vi "Actor Core.vi"(8 "error in":errorcluster, 11 "Pane Relief Main UI in":refnum<class "Pane Relief Main UI.lvclass">) -> (0 "error out":errorcluster, 3 "Actor out":refnum<class "Actor.lvclass">)   [LabVIEW 2018, in "Pane Relief Main UI.lvlib" / "Pane Relief Main UI.lvclass"]
uses:
  <resource>/dialog/QuickDrop/plugins/PaneRelief/Classes/Pane Relief Main UI/Pane Relief Main UI/Pane Relief Main UI.lvclass
  C:/Program Files (x86)/National Instruments/LabVIEW 2018/vi.lib/MGI/Panel Manager/Panel Actor/Panel Actor/Panel Actor.lvclass
  <vilib>/ActorFramework/Actor/Actor.lvclass
  <resource>/dialog/QuickDrop/plugins/PaneRelief/Classes/Splitter Settings UI/Splitter Settings UI/Splitter Settings UI.lvclass
  <resource>/dialog/QuickDrop/plugins/PaneRelief/Classes/Pane Settings UI/Pane Settings UI/Pane Settings UI.lvclass
  <resource>/dialog/QuickDrop/plugins/PaneRelief/Classes/Pane Relief Main UI/Pane Relief Main UI/Pane Relief Main UI.lvclass/Pane Relief Main UI.ctl
  <vilib>/ActorFramework/Message Enqueuer/Message Enqueuer.lvclass/Message Enqueuer.ctl
  <resource>/dialog/QuickDrop/plugins/PaneRelief/Typedefs/UI Selections--Cluster.ctl
  <resource>/dialog/QuickDrop/plugins/PaneRelief/Typedefs/Point--Cluster.ctl
  <vilib>/Utility/sysdir.llb/System Directory Type.ctl
  <resource>/dialog/QuickDrop/plugins/PaneRelief/Classes/Panel Object/Panel Object.lvclass
  <resource>/dialog/QuickDrop/plugins/PaneRelief/Typedefs/Selection Colors--Cluster.ctl
  <vilib>/ActorFramework/Message Enqueuer/Enqueue.vi
  <vilib>/MGI/Panel Manager/Panel/Panel/Subpanel/Subpanel.lvclass
  C:/Program Files (x86)/National Instruments/LabVIEW 2018/vi.lib/MGI/Panel Manager/Panel/Panel/Panel.lvclass
  <vilib>/ActorFramework/Stop Msg/Stop Msg.lvclass
  C:/Program Files (x86)/National Instruments/LabVIEW 2018/vi.lib/ActorFramework/Message/Message.lvclass
  <resource>/dialog/QuickDrop/plugins/PaneRelief/Classes/Splitter/Splitter.lvclass
  C:/Program Files (x86)/National Instruments/LabVIEW 2018/resource/dialog/QuickDrop/plugins/PaneRelief/Classes/Panel Object/Panel Object.lvclass
  <resource>/dialog/QuickDrop/plugins/PaneRelief/Classes/Pane/Pane.lvclass
  <vilib>/MGI/Panel Manager/Panel/Panel/Subpanel/Subpanel.vi
  <vilib>/ActorFramework/Message Priority Queue/Priority Enqueue.vi
  <vilib>/MGI/Panel Manager/Panel Actor/Panel Actor/Panel Actor.lvclass
  <vilib>/MGI/Panel Manager/Panel/Panel.lvlib
panel:
  out "Nav Pic":picture
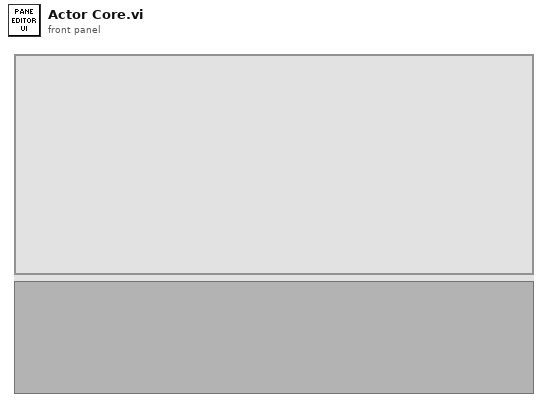
[diagram p1: front panel]
types:
  T1 = cluster{"Pnl Actor":refnum<event-registration>, "Event Registration Refnum":refnum<event-registration>}
  T2 = enum32{"Invalid", "Standard", "Closed", "Hidden", "Minimized", "Maximized"}
  T3 = enum32{"invalid app kind", "Development System", "Run Time System", "Student Edition", "Embedded LabVIEW", "Evaluation", "Custom"}
  T4 = typedef "LVPoint32TypeDef.ctl" = cluster{"Horizontal":i32, "Vertical":i32}
  T5 = typedef "Point--Cluster.ctl" = cluster{"Horizontal":i32, "Vertical":i32}
  T6 = typedef "UI Selections--Cluster.ctl" = cluster{"Mouse-over Idx":i32, "Selected Idx":i32}
  T7 = cluster{"Core":cluster{"Current VI Reference":refnum<vi>, "Close Panel on Exit?":bool}, "QD Launch VI Ref":refnum<vi>, "Panel Objects[]":refnum<class "Panel Object.lvclass">[], "UI Selections":T6, "Scale Factor":dbl, "Nav Pic Offset":T5, "Persistent Data Folder":path, "Persistent Data File":string}
  T8 = typedef "System Directory Type.ctl" = i32
  T9 = cluster{"Current VI Reference":refnum<vi>, "Close Panel on Exit?":bool}
  T10 = typedef "LVBoundsTypeDef.ctl" = cluster{"Width":u32, "Height":u32}
  T11 = typedef "LVPointTypeDef.ctl" = cluster{"Horizontal":i16, "Vertical":i16}
  T12 = typedef "Selection Colors--Cluster.ctl" = cluster{"Normal":u32, "Mouse-over":u32, "Selected":u32}
  T13 = typedef "imagedata.ctl" = cluster{"image type":i32, "image depth":i32, "image":u8[], "mask":u8[], "colors":u32[], "Rectangle":cluster{"left":i16, "top":i16, "right":i16, "bottom":i16}}
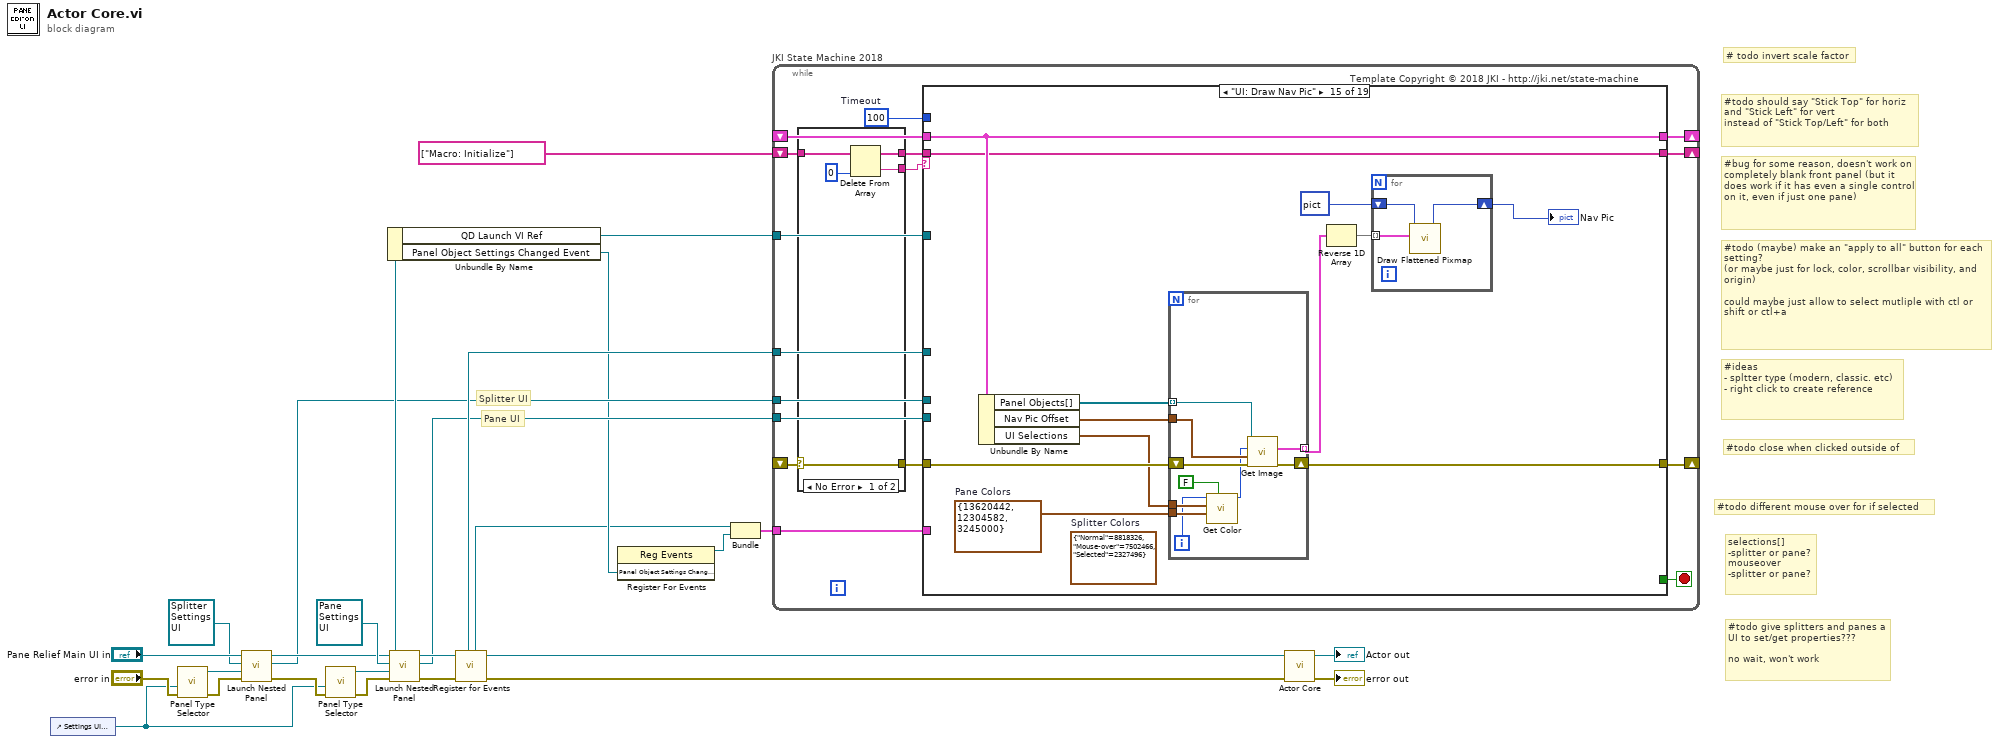
[diagram p0: block diagram]
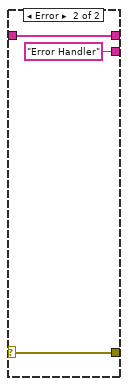
[diagram p2: hidden frame]
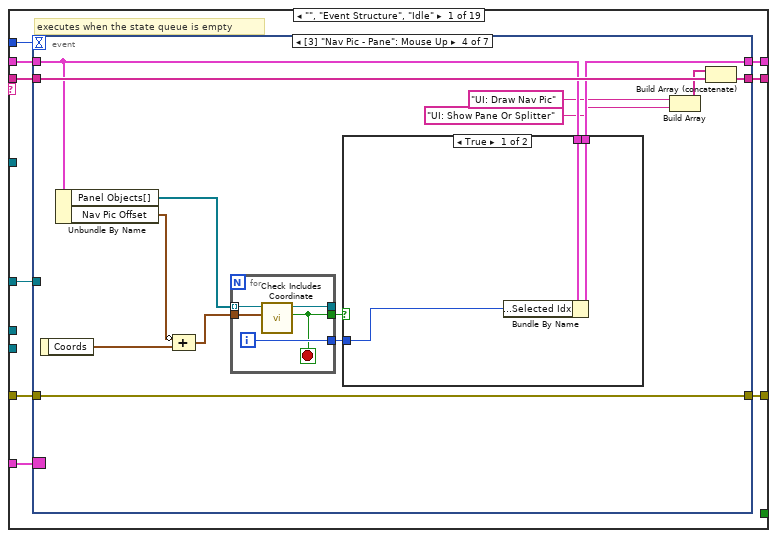
[diagram p3: hidden frame]
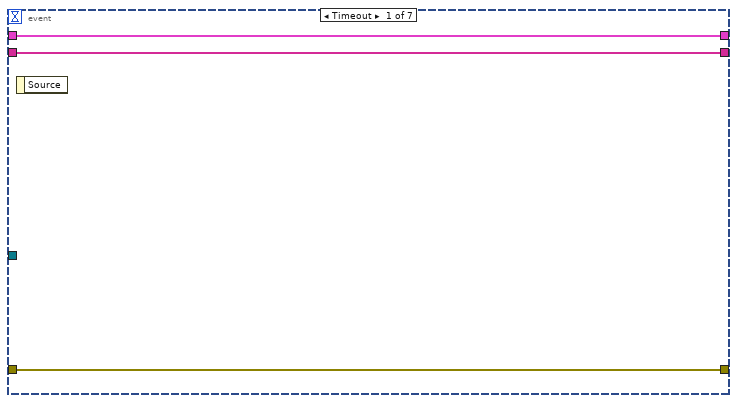
[diagram p4: hidden frame]
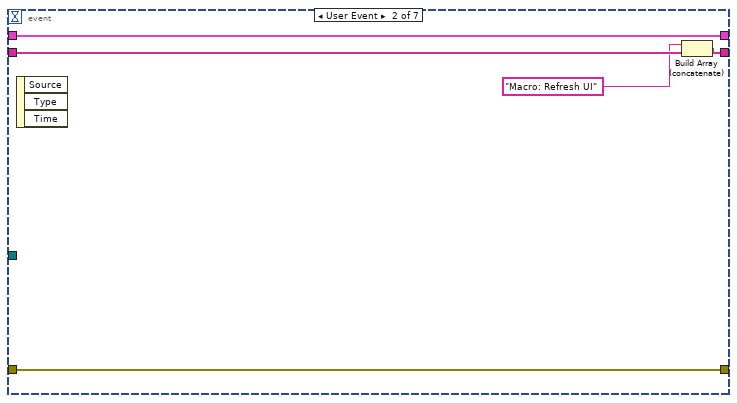
[diagram p5: hidden frame]
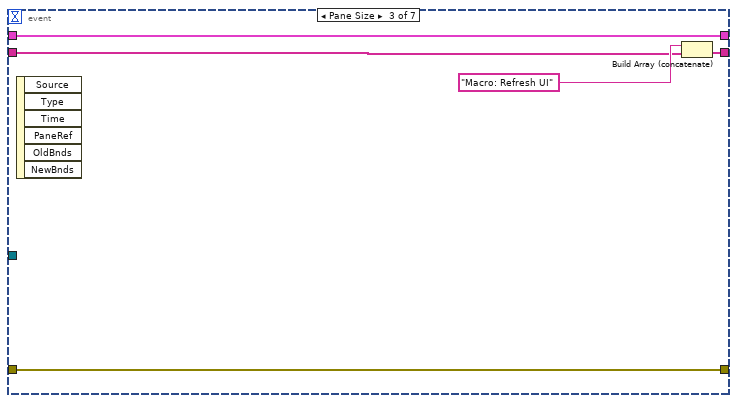
[diagram p6: hidden frame]
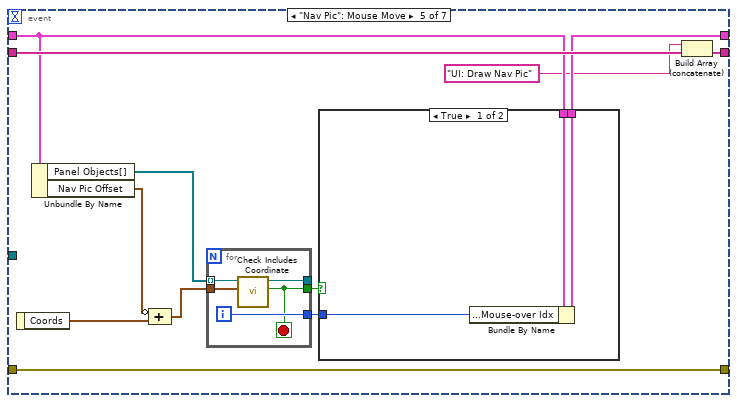
[diagram p8: hidden frame]
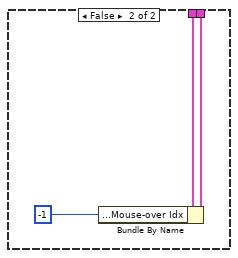
[diagram p9: hidden frame]
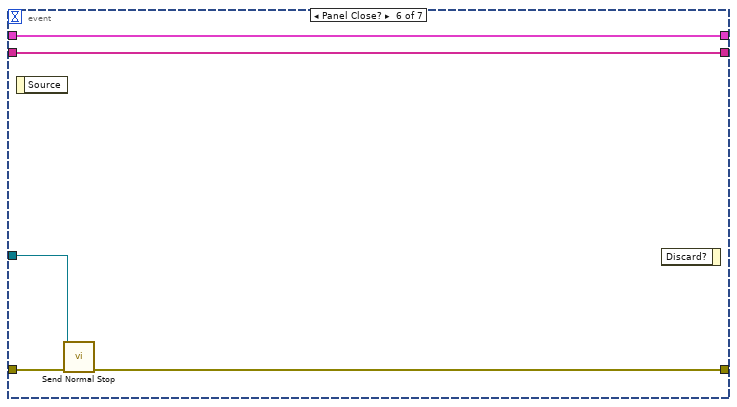
[diagram p10: hidden frame]
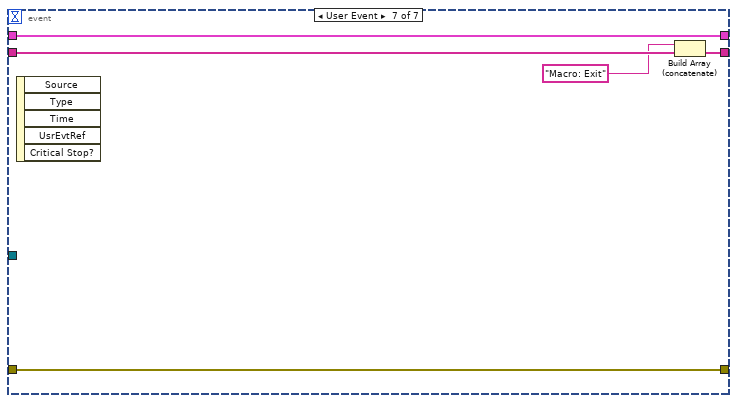
[diagram p11: hidden frame]
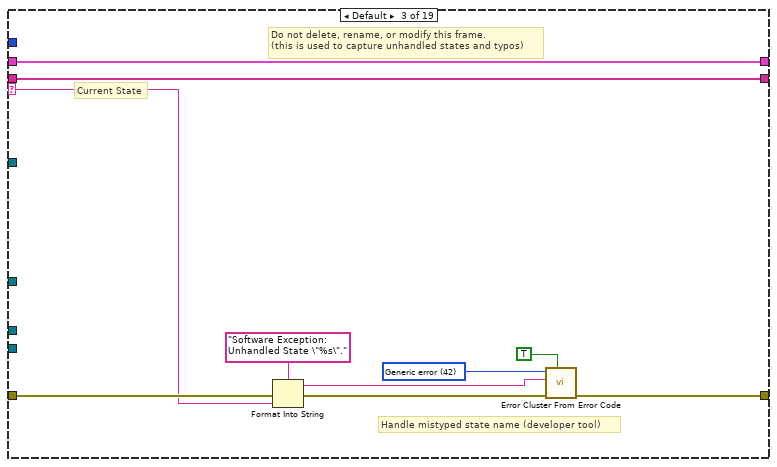
[diagram p13: hidden frame]
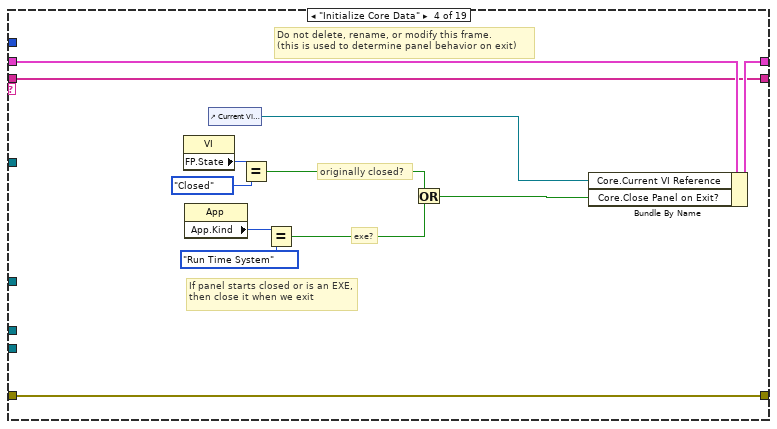
[diagram p14: hidden frame]
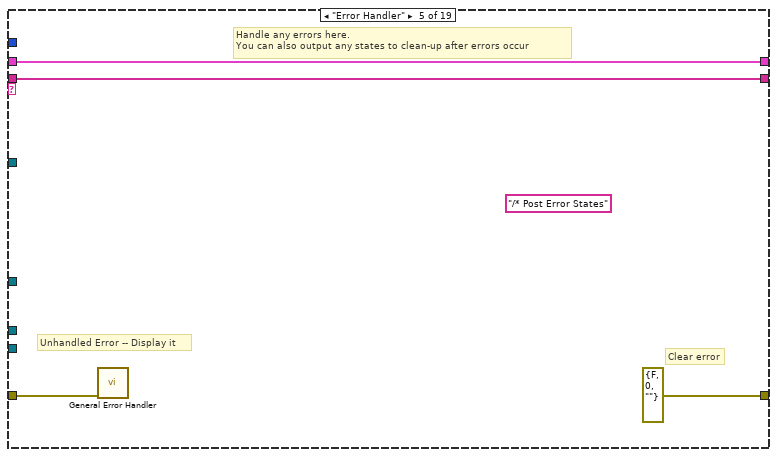
[diagram p15: hidden frame]
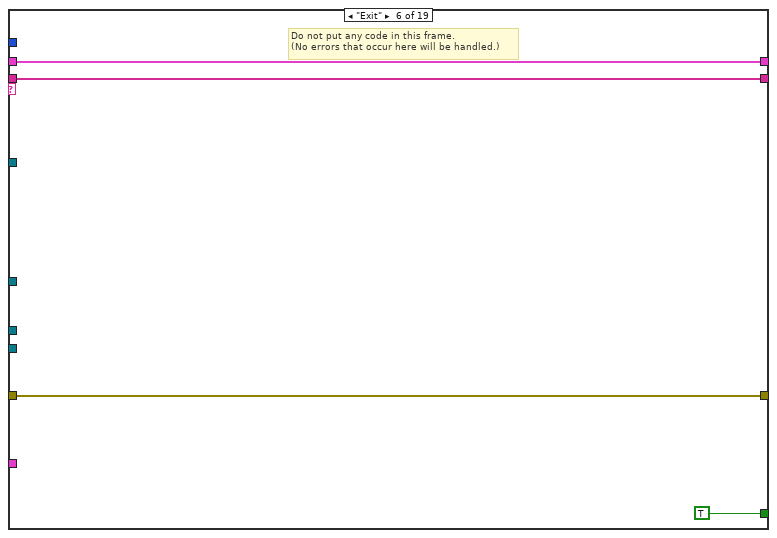
[diagram p16: hidden frame]
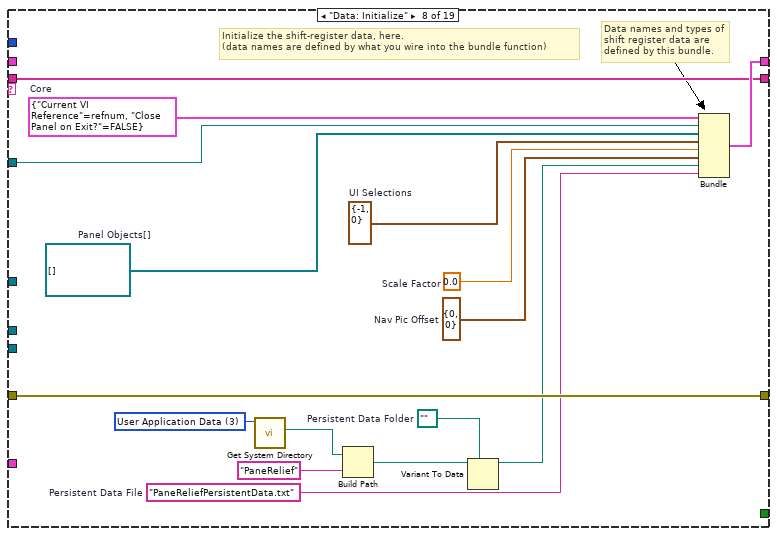
[diagram p18: hidden frame]
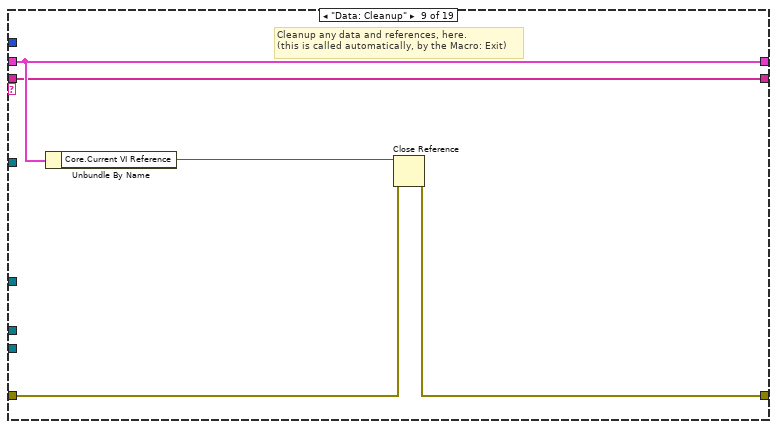
[diagram p19: hidden frame]
diagram:
  # "Pane UI"
  # "Splitter UI"
  # "#todo close when clicked outside of"
  # "#todo give splitters and panes a UI to set/get properties???\n\nno wait, won't work"
  # "# todo invert scale factor"
  # "selections[]\n-splitter or pane?\nmouseover\n-splitter or pane?"
  # "#todo different mouse over for if selected"
  # "#ideas\n- spltter type (modern, classic. etc)\n- right click to create reference"
  # "#todo (maybe) make an \"apply to all\" button for each setting?\n(or maybe just for lock, color, scrollbar visibility, and origin)\n\ncould maybe just allow to select mutliple with ctl or shift or ctl+a"
  # "#todo should say \"Stick Top\" for horiz and \"Stick Left\" for vert\ninstead of \"Stick Top/Left\" for both"
  # "#bug for some reason, doesn't work on completely blank front panel (but it does work if it has even a single control on it, even if just one pane)"
  n1 = control-ref of="Settings UI Subpanel"() -> (w12:refnum<vi>)
  n2 = call-poly <vilib>:"Panel Type Selector.vi"("Error In"="error in", "Sub Panel"=w12) -> ("Error Out"=w19:errorcluster, "Subpanel Out"=w22:refnum<class "Subpanel.lvclass">)  [unwired: 8 in]
  n3 = call <vilib>:"Launch Nested Panel.vi"("error in (no error)"=w19, "Panel"=w22, "Nested Panel Actor"=refnum<class "Splitter Settings UI.lvclass"> refnum ("Splitter Settings UI.lvlib:Splitter Settings UI.lvclass"), "Panel Actor in"="Pane Relief Main UI in") -> ("error out"=w13:errorcluster, "Nested Actor's Enqueuer"=w6:refnum<class "Message Enqueuer.lvclass">, "Panel Actor out"=w14:refnum<class "Pane Relief Main UI.lvclass">)  [unwired: 4 in, 1 out]
  n4 = call-poly <vilib>:"Panel Type Selector.vi"("Error In"=w13, "Sub Panel"=w12) -> ("Error Out"=w16:errorcluster, "Subpanel Out"=w15:refnum<class "Subpanel.lvclass">)  [unwired: 8 in]
  n5 = call <vilib>:"Launch Nested Panel.vi"("error in (no error)"=w16, "Panel"=w15, "Nested Panel Actor"=refnum<class "Pane Settings UI.lvclass"> refnum ("Pane Settings UI.lvlib:Pane Settings UI.lvclass"), "Panel Actor in"=w14) -> ("error out"=w9:errorcluster, "Nested Actor's Enqueuer"=w5:refnum<class "Message Enqueuer.lvclass">, "Panel Actor out"=w11:refnum<class "Pane Relief Main UI.lvclass">)  [unwired: 4 in, 1 out]
  n6 = Unbundle By Name(w11) -> ("QD Launch VI Ref"=w23:refnum<vi>, "Panel Object Settings Changed Event"=w4:refnum<user-event>)
  n7 = call <vilib>:"Register for Events.vi"("Error In"=w9, "Panel Actor in"=w11) -> ("Error Out"=w8:errorcluster, "Panel Actor out"=w10:refnum<class "Pane Relief Main UI.lvclass">, "Pnl Actor"=w3:refnum<event-registration>, "Self Enqueuer"=w7:refnum<class "Message Enqueuer.lvclass">)  [unwired: 6 in]
  n8 = register-events(w4) -> (reference out=w1:refnum<event-registration>)  [unwired: 2 in, 1 out]
  n9 = Bundle("Pnl Actor"=w3, "Event Registration Refnum"=w1) -> (w2:T1)  [unwired: 1 in]
  n10 = while "JKI State Machine 2018" {
    shift-right: [w39] -> _
    shift-left: _ -> [w38]
    shift-right: [w42] -> _
    shift-left: _ -> [w32]
    shift-right: [w41] -> _
    shift-left: string[] ["Macro: Initialize"] -> [w36]
    tunnel: w23 -> [w31]
    tunnel: w2 -> [w30]
    tunnel: w7 -> [w27]
    tunnel: w6 -> [w29]
    tunnel: w5 -> [w28]
    stop <- w40 stop-if-true
    w37 = 100  # Timeout
    # "Template Copyright © 2018 JKI - http://jki.net/state-machine"
    n11 = case shown="No Error" w32 {
      selector: w32 -> [w43 w50]
      tunnel: w36 -> [w47 w49]
      tunnel: [w46 w49] -> w35
      tunnel: [w45 "Error Handler" ("String")] -> w34
      tunnel: [w43 w50] -> w33
      frame No Error {
        n12 = Delete From Array(array=w47, index=0) -> (deleted portion=w45:string, array with subset deleted=w46:string[])  [unwired: 1 in]
      }
      frame Error {
      }
    }
    n13 = case shown="\"UI: Draw Nav Pic\"" w34 {
      selector: w34 -> [_ _ w135 _ _ _ _ _ _ _ _ _ _ _ _ _ _ _ _]
      tunnel: w35 -> [w59 w129 w132 w142 w154 w158 w162 w167 w181 w186 w189 w197 w199 w230 w263 w278 w283 w288 w293]
      tunnel: w38 -> [w57 w130 w136 w148 w156 w161 w163 _ w182 w187 w191 w198 w206 w234 w264 w279 w284 w289 w294]
      tunnel: [w56 w131 w138 w152 errorcluster {"status"=FALSE, "code"=0, "source"=""} ("error out") w160 w164 w179 w183 w188 w190 w193 w203 w233 w254 w280 w285 w290 w295] -> w42
      tunnel: w33 -> [w53 w131 w137 w152 w155 w160 w164 w179 w184 w188 w190 w194 w211 w236 w262 w280 w285 w290 w295]
      tunnel: [w58 w129 w132 w142 w154 w158 w162 w167 w181 w186 w189 w197 w199 w230 w263 w278 w281 w286 w292] -> w41
      tunnel: [_ _ _ _ _ TRUE _ _ _ _ _ _ _ _ _ _ _ _ _] -> w40
      tunnel: [w55 w130 w136 w153 w156 w161 w163 w180 w182 w187 w191 w198 w201 w235 w264 w279 w284 w289 w294] -> w39
      tunnel: w37 -> [w54 _ _ _ _ _ _ _ _ _ _ _ _ _ _ _ _ _ _]
      tunnel: w31 -> [_ _ _ _ _ _ _ w165 _ _ _ _ _ _ _ _ _ _ _]
      tunnel: w30 -> [w52 _ _ _ _ _ _ _ _ _ _ _ _ _ _ _ _ _ _]
      tunnel: w29 -> [_ _ _ _ _ _ _ _ _ _ _ _ _ w219 _ _ _ _ _]
      tunnel: w28 -> [_ _ _ _ _ _ _ _ _ _ _ _ _ w218 _ _ _ _ _]
      tunnel: w27 -> [w51 _ _ _ _ _ _ _ _ _ _ _ _ _ _ _ _ _ _]
      frame "", "Event Structure", "Idle" {
        # "executes when the state queue is empty"
        n14 = event shown="[3] \"Nav Pic - Pane\": Mouse Up" {
          selector: w52 -> [_ _ _ _ _ _ _]
          dyn-events: _ -> [_ _ _ _ _ _ _]
          timeout: w54 -> [_ _ _ _ _ _ _]
          tunnel: w59 -> [w60 w65 w69 w86 w107 w119 w126]
          tunnel: [w60 w64 w68 w85 w106 w119 w124] -> w58
          tunnel: w57 -> [w61 w66 w71 w82 w103 w123 w127]
          tunnel: [w62 w67 w72 w84 w105 w121 w128] -> w56
          tunnel: [w61 w66 w71 w83 w104 w123 w127] -> w55
          tunnel: w53 -> [w62 w67 w72 w84 w105 w120 w128]
          tunnel: w51 -> [_ _ _ _ _ w122 _]
          event Timeout {
            n15 = event-data() -> ()  [unwired: 1 in, 1 out]
          }
          event User Event {
            n16 = event-data() -> ()  [unwired: 1 in, 3 out]
            n17 = Build Array (concatenate)("Macro: Refresh UI" ("State(s) in Front (\"\")"), w65) -> (w64:string[])
          }
          event Pane Size {
            n18 = event-data() -> ()  [unwired: 1 in, 6 out]
            n19 = Build Array (concatenate)("Macro: Refresh UI", w69) -> (w68:string[])
          }
          event Mouse Up {
            n20 = event-data() -> ("Coords"=w77:T4)  [unwired: 1 in]
            n21 = Unbundle By Name(w82) -> ("Panel Objects[]"=w75:refnum<class "Panel Object.lvclass">[], "Nav Pic Offset"=w78:T5)
            n22 = Compound Arithmetic op=ADD(invert w78, w77) -> (w74:T5)
            n23 = for {
              tunnel: [w91] -> _
              tunnel: [w87] -> w81
              tunnel: w75 -> [w90] mode=indexing
              tunnel: w74 -> [w89]
              tunnel: [w88] -> w73
              i -> [w88]
              stop <- w87 stop-if-true
              n24 = call-dynamic "Check Includes Coordinate.vi"("Coordinate"=w89, "Panel Object in"=w90) -> ("Included?"=w87:bool, "Panel Object out"=w91:refnum<class "Panel Object.lvclass">)  [unwired: 7 in, 1 out]
            }
            n25 = case shown="True" w81 {
              tunnel: [w94 w95] -> w83
              tunnel: w82 -> [w93 w95]
              tunnel: w73 -> [w92 _]
              frame True {
                n26 = Bundle By Name(cluster=w93, "UI Selections.Selected Idx"=w92) -> (w94:T7)
              }
              frame False {
              }
            }
            n27 = Build Array("UI: Draw Nav Pic", "UI: Show Pane Or Splitter") -> (w79:string[])
            n28 = Build Array (concatenate)(w79, w86) -> (w85:string[])
          }
          event "Nav Pic": Mouse Move {
            n29 = event-data() -> ("Coords"=w100:T4)  [unwired: 1 in]
            n30 = Unbundle By Name(w103) -> ("Panel Objects[]"=w99:refnum<class "Panel Object.lvclass">[], "Nav Pic Offset"=w101:T5)
            n31 = Compound Arithmetic op=ADD(invert w101, w100) -> (w98:T5)
            n32 = for {
              tunnel: [w112] -> _
              tunnel: [w108] -> w102
              tunnel: w99 -> [w111] mode=indexing
              tunnel: w98 -> [w110]
              tunnel: [w109] -> w97
              i -> [w109]
              stop <- w108 stop-if-true
              n33 = call-dynamic "Check Includes Coordinate.vi"("Coordinate"=w110, "Panel Object in"=w111) -> ("Included?"=w108:bool, "Panel Object out"=w112:refnum<class "Panel Object.lvclass">)  [unwired: 7 in, 1 out]
            }
            n34 = case shown="True" w102 {
              tunnel: [w115 w118] -> w104
              tunnel: w103 -> [w114 w117]
              tunnel: w97 -> [w113 _]
              frame True {
                n35 = Bundle By Name(cluster=w114, "UI Selections.Mouse-over Idx"=w113) -> (w115:T7)
              }
              frame False {
                n36 = Bundle By Name(cluster=w117, "UI Selections.Mouse-over Idx"=-1) -> (w118:T7)
              }
            }
            n37 = Build Array (concatenate)("UI: Draw Nav Pic", w107) -> (w106:string[])
          }
          event Panel Close? {
            n38 = event-data() -> ()  [unwired: 1 in, 1 out]
            n39 = call <vilib>:"Send Normal Stop.vi"("error in (no error)"=w120, "Message Enqueuer"=w122) -> ("error out"=w121:errorcluster)  [unwired: 9 in]
            n40 = event-data() -> ()  [unwired: 2 in, 1 out]
          }
          event User Event {
            n41 = event-data() -> ()  [unwired: 1 in, 5 out]
            n42 = Build Array (concatenate)("Macro: Exit", w126) -> (w124:string[])
          }
        }
      }
      frame "---------- Core ----------" {
        # "Do not put any code in this frame.\n(it is a separator no-op)"
      }
      frame Default {
        w134 = 42 items=["No error", "Argument error", "Memory is full", "Out of zone", "End of file", "File already open", "Generic file I/O error", "File not found", "File permission error", "Disk is full", "Duplicate path", "Too many files open", "System feature not enabled", "Resource file not found", "Cannot add resource", "Resource not found", "Image not found", "Image memory error", "Pen does not exist", "Config type invalid", "Config token not found", "Config parse error", "Config memory error", "Bad external code format", "Bad external code offset", "External code not present", "Null window", "Destroy window error", "Null menu", "Print aborted", "Bad print record", "Print driver error", "Windows error during printing", "Memory error during printing", "Print dialog error", "Generic print error", "Invalid device refnum", "Device not found", "Device parameter error", "Device unit error", "Cannot open device", "Device call aborted", "Generic error", "Cancelled by user", "Object ID too low", "Object ID too high", "Object not in heap", "Unknown heap", "Unknown object (invalid DefProc)", "Unknown object (DefProc not in table)", "Message out of range", "Invalid (null) method", "Unknown message", "Manager call not supported", "Bad address", "Network operation in progress", "Network operation timed out", "Connection is busy", "Network attribute not supported", "Network error", "Address in use", "System out of memory", "Connection aborted", "Connection refused", "Not connected", "Already connected", "Connection closed", "Initialization error (interapplication manager)", "Bad occurrence", "Wait on unbound occurrence handler", "Occurrence queue overflow", "Datalog type conflict", "Unused", "Unrecognized type (interapplication manager)", "Memory corrupt", "Failed to make temporary DLL", "Old CIN version", "Drag socket not found", "Failed to load drop-object", "Failed to register OLE object", "Failed to release OLE object", "Format specifier type mismatch", "Unknown format specifier", "Too few format specifiers", "Too many format specifiers", "Scan failed", "Newer CIN version", "Error converting to variant", "Runtime menu error", "Password tampered", "Variant attribute not found", "Incompatible variant data type", "Event data is not available", "Event Store is not present", "Occurrence is not found", "Event Queue is not created", "Event info is not available", "Refnum passed is NULL", "Error retrieving Class GUID", "Error retrieving CoClass GUID", "Error retrieving TypeLib GUID.", "Bad built application magic bytes.", "Specific driver is different from the specific driver associated with the Logical Name.", "There is no session opened to the class driver.", "Max Error", "MAX - Error with config objects", "MAX - Error loading configuration", "MAX - Group not supported"]
        # "Current State"
        # "Do not delete, rename, or modify this frame.\n(this is used to capture unhandled states and typos)"
        # "Handle mistyped state name (developer tool)"
        n43 = Format Into String(format string="Software Exception: Unhandled State \"%s\"." ("message"), error in=w137, w135) -> (resulting string=w140:string, error out=w139:errorcluster)  [unwired: 1 in]
        n44 = call <vilib>:"Error Cluster From Error Code.vi"("show call chain? (False)"=TRUE, "error in (no error)"=w139, "error message (\"\")"=w140, "error code (0)"=w134) -> ("error out"=w138:errorcluster)  [unwired: 5 in]
      }
      frame "Initialize Core Data" {
        # "Do not delete, rename, or modify this frame.\n(this is used to determine panel behavior on exit)"
        # "originally closed?"
        # "exe?"
        # "If panel starts closed or is an EXE, then close it when we exit"
        n45 = property class="VI"() -> ("FP.State"=w145:T2)  [unwired: 2 in, 2 out]
        n46 = property class="App"() -> ("App.Kind"=w151:T3)  [unwired: 2 in, 2 out]
        n47 = control-ref of="Current VI Reference"() -> (w146:refnum<vi>)
        n48 = Equal?(x=w145, y=T2."Closed" ("Front Panel Window:State")) -> (x = y?=w143:bool)
        n49 = Equal?(x=w151, y=T3."Run Time System" ("Application:Kind")) -> (x = y?=w149:bool)
        n50 = Or(x=w143, y=w149) -> (x .or. y?=w147:bool)
        n51 = Bundle By Name(cluster=w148, "Core.Current VI Reference"=w146, "Core.Close Panel on Exit?"=w147) -> (w153:T7)
      }
      frame "Error Handler" {
        (unwired) "/* Post Error States"
        # "Unhandled Error -- Display it"
        # "Handle any errors here.\nYou can also output any states to clean-up after errors occur"
        # "Clear error"
        n52 = call <vilib>:"General Error Handler.vi"("error in (no error)"=w155) -> ()  [unwired: 10 in, 5 out]
      }
      frame "Exit" {
        # "Do not put any code in this frame.\n(No errors that occur here will be handled.)"
      }
      frame "---------- Data ----------" {
        # "Do not put any code in this frame.\n(It is a separator no-op. You can make a copy of this frame to create a new Data frame)"
      }
      frame "Data: Initialize" {
        w166 = refnum<class "Panel Object.lvclass">[] []  # Panel Objects[]
        w171 = path ""  # Persistent Data Folder
        w168 = "PaneReliefPersistentData.txt"  # Persistent Data File
        w174 = T8 3 items=["User Home"=0, "User Desktop"=1, "User Documents"=2, "User Application Data"=3, "User Preferences"=4, "User Temporary"=5, "Public Documents"=6, "Public Application Data"=7, "Public Preferences"=8, "Public Cache"=13, "System Core Libraries"=9, "System Installed Libraries"=10, "Application Files"=11, "Boot Volume Root"=12] ("system directory type")
        w175 = T5 {"Horizontal"=0, "Vertical"=0}  # Nav Pic Offset
        w176 = 0.0  # Scale Factor
        w177 = T6 {"Mouse-over Idx"=-1, "Selected Idx"=0}  # UI Selections
        w178 = T9 {"Current VI Reference"=refnum, "Close Panel on Exit?"=FALSE}  # Core
        # "Data names and types of shift register data are defined by this bundle."
        # "Initialize the shift-register data, here.\n(data names are defined by what you wire into the bundle function)"
        n53 = call <vilib>:"Get System Directory.vi"("system directory type"=w174) -> ("system directory"=w172:path)  [unwired: 10 in]
        n54 = Build Path(base path=w172, name or relative path="PaneRelief") -> (appended path=w169:path)
        n55 = Variant To Data(type=w171, Variant=w169) -> (data=w170:path)  [unwired: 1 in, 1 out]
        n56 = Bundle("Core"=w178, "QD Launch VI Ref"=w165, "Panel Objects[]"=w166, "UI Selections"=w177, "Scale Factor"=w176, "Nav Pic Offset"=w175, "Persistent Data Folder"=w170, "Persistent Data File"=w168) -> (w180:T7)  [unwired: 1 in]
      }
      frame "Data: Cleanup" {
        # "Cleanup any data and references, here.\n(this is called automatically, by the Macro: Exit)"
        n57 = Unbundle By Name(w182) -> ("Core.Current VI Reference"=w185:refnum<vi>)
        n58 = Close Reference(reference=w185, error in (no error)=w184) -> (error out=w183:errorcluster)
      }
      frame "---------- UI ----------" {
        # "Do not put any code in this frame.\n(It is a separator no-op. You can make a copy of this frame to create a new UI frame)"
      }
      frame "UI: Initialize" {
        # "Initialize the User Interface, here.\n(this is called automatically, by the Macro: Init)"
      }
      frame "UI: Show Pane Or Splitter" {
        n59 = Unbundle By Name(w198) -> ("Panel Objects[]"=w196:refnum<class "Panel Object.lvclass">[], "UI Selections.Selected Idx"=w195:i32)
        n60 = Index Array(array=w196, index=w195) -> (element=w192:refnum<class "Panel Object.lvclass">)
        n61 = call-dynamic "Show Settings UI.vi"("Error In"=w194, "Panel Object in"=w192) -> ("Error Out"=w193:errorcluster)  [unwired: 8 in, 1 out]
      }
      frame "UI: Calculate Scale Factor" {
        # "#todo doesn't give right area if VI is empty"
        n62 = Unbundle By Name(w206) -> ("QD Launch VI Ref"=w209:refnum<vi>)
        n63 = property class="VI"(reference=w209, error in=w211) -> (error out=w213:errorcluster, "Panel"=w212:refnum<vi>)  [unwired: 1 out]
        n64 = property class="Pnl"(reference=w212, error in=w213) -> (error out=w208:errorcluster, "Width"=w210:u32, "Height"=w214:u32)  [unwired: 1 out]
        n65 = property on="Nav Pic" class="Pict"(error in=w208) -> (error out=w203:errorcluster, "Draw Area Size"=w207:T10)  [unwired: 1 in, 1 out]
        n66 = Unbundle By Name(w207) -> ("Width"=w205:u32, "Height"=w204:u32)
        n67 = call <resource>:"Calculate Scaling Factors.vi"("Max Picture Size Y"=w204, "Max Picture Size X"=w205, "Panel Height"=w214, "Panel Width"=w210) -> ("Scale Factor"=w202:dbl, "Offset (to center)"=w200:T5)  [unwired: 6 in]
        n68 = Bundle By Name(cluster=w206, "Nav Pic Offset"=w200, "Scale Factor"=w202) -> (w201:T7)
      }
      frame "UI: Get Pane And Splitter Details" {
        n69 = Unbundle By Name(w234) -> ("Scale Factor"=w231:dbl, "QD Launch VI Ref"=w225:refnum<vi>)
        n70 = property class="VI"(reference=w225, error in=w236) -> (error out=w238:errorcluster, "Panel"=w237:refnum<vi>)  [unwired: 1 out]
        n71 = property class="Pnl"(reference=w237, error in=w238) -> (error out=w224:errorcluster, "Panes[]"=w217:refnum<vi>[], "Splitters[]"=w226:refnum<vi>[])  [unwired: 1 out]
        n72 = Index Array(array=w217) -> (element=w221:refnum<vi>)  [unwired: 1 in]
        n73 = property class="Pane"(reference=w221, error in=w224) -> (reference out=w229:refnum<vi>, error out=w228:errorcluster, "Origin"=w227:T11)
        n74 = invoke on="Invoke Node" class="Pane" method="CvtPaneToPanelCoords"(reference=w229, error in=w228, "PaneCoords"=w227) -> (error out=w223:errorcluster, "PanelCoords"=w222:T11)  [unwired: 2 in, 3 out]
        n75 = for {
          tunnel: w231 -> [w250]
          tunnel: w217 -> [w249] mode=indexing
          shift-right: [w251] -> w232
          shift-left: w223 -> [w252]
          tunnel: [w248] -> w215 mode=indexing
          tunnel: w222 -> [w247]
          tunnel: w218 -> [w246]
          n76 = call <resource>:"Pane.vi"("Settings UI Enqueuer"=w246, "Error In"=w252, "Offset"=w247, "Scale Factor"=w250, "Pane Ref"=w249) -> ("Error Out"=w251:errorcluster, "Pane out"=w248:refnum<class "Pane.lvclass">)  [unwired: 5 in]
        }
        n77 = for {
          tunnel: w231 -> [w243]
          tunnel: w226 -> [w242] mode=indexing
          shift-right: [w245] -> w233
          shift-left: w232 -> [w244]
          tunnel: [w241] -> w216 mode=indexing
          tunnel: w222 -> [w240]
          tunnel: w219 -> [w239]
          n78 = call <resource>:"Splitter.vi"("Settings UI Enqueuer"=w239, "Error In"=w244, "Offset"=w240, "Scale Factor"=w243, "Splitter Ref"=w242) -> ("Error Out"=w245:errorcluster, "Splitter out"=w241:refnum<class "Splitter.lvclass">)  [unwired: 5 in]
        }
        n79 = Build Array (concatenate)(w216, w215) -> (w220:refnum<class "Panel Object.lvclass">[])
        n80 = Bundle By Name(cluster=w234, "Panel Objects[]"=w220) -> (w235:T7)
      }
      frame "UI: Draw Nav Pic" {
        (unwired) T12 {"Normal"=8818326, "Mouse-over"=7502466, "Selected"=2327496}  # Splitter Colors
        w259 = T12 {"Normal"=13620442, "Mouse-over"=12304582, "Selected"=3245000}  # Pane Colors
        n81 = Unbundle By Name(w264) -> ("Panel Objects[]"=w258:refnum<class "Panel Object.lvclass">[], "Nav Pic Offset"=w260:T5, "UI Selections"=w261:T6)
        n82 = for {
          tunnel: w260 -> [w277]
          shift-right: [w275] -> w254
          shift-left: w262 -> [w276]
          tunnel: w261 -> [w274]
          tunnel: w258 -> [w273] mode=indexing
          tunnel: w259 -> [w271]
          tunnel: [w268] -> w257 mode=indexing
          i -> [w269]
          n83 = call <resource>:"Get Color.vi"("Splitter? (F: Pane)"=FALSE, "Pane Colors"=w271, "UI Selections"=w274, "Item Index"=w269) -> ("Color"=w270:u32)  [unwired: 7 in]
          n84 = call-dynamic "Get Image.vi"("Error In"=w276, "Offset"=w277, "Color Box"=w270, "Panel Object in"=w273) -> ("Error Out"=w275:errorcluster, "Image"=w268:T13)  [unwired: 5 in, 1 out]
        }
        n85 = Reverse 1D Array(array=w257) -> (reversed array=w253:T13[])
        n86 = for {
          tunnel: w253 -> [w267] mode=indexing
          shift-right: [w265] -> w256
          shift-left: picture data[5B] ("new picture") -> [w266]
          n87 = call <vilib>:"Draw Flattened Pixmap.vi"("image data"=w267, "picture"=w266) -> ("new picture"=w265:picture)  [unwired: 7 in]
        }
        "Nav Pic" <- w256
      }
      frame "---------- Macro ----------" {
        # "Do not put any code in this frame.\n(It is a separator no-op. You can make a copy of this frame to create a new Macro frame)"
      }
      frame "Macro: Initialize" {
        # "Initialization Macro\n(This is called once, when the VI starts)"
        n88 = Build Array (concatenate)(string[] ["Data: Initialize", "Initialize Core Data", "Macro: Refresh UI", "UI: Initialize", "UI: Show Pane Or Splitter"], w283) -> (w281:string[])
      }
      frame "Macro: Refresh UI" {
        n89 = Build Array (concatenate)(string[] ["UI: Calculate Scale Factor", "UI: Get Pane And Splitter Details", "UI: Draw Nav Pic"], w288) -> (w286:string[])
      }
      frame "Macro: Exit" {
        # "Exit Macro\n(This is called once, when the VI exits)"
        n90 = Unbundle By Name(w294) -> ()  [unwired: 1 out]
        n91 = Build Array (concatenate)(string[] ["Data: Cleanup", "Exit"], w293) -> (w292:string[])
      }
    }
  }
  n92 = call-parent "Actor Core.vi"("error in"=w8, "Panel Actor in"=w10) -> ("error out"=→"error out":errorcluster, "Actor out"=→"Actor out":refnum<class "Actor.lvclass">)  [unwired: 8 in]
